vi "3dtest.vi"() -> ()   [LabVIEW 2022 SP3]
panel:
  in  "Planes to insert":u8=1
  in  "Save to File?":bool
  out "Array":u8[][][](array[numeric])
  in  "8-bit pixmap":u8[][][](array[numeric])=array17x236x252[1011024 elements]
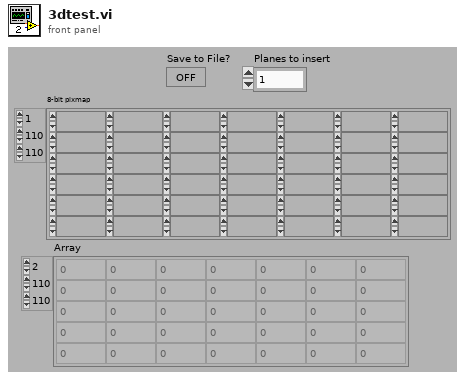
[diagram p1: front panel]
types:
  T1 = enum16{"open", "open or create", "create or replace", "create"}
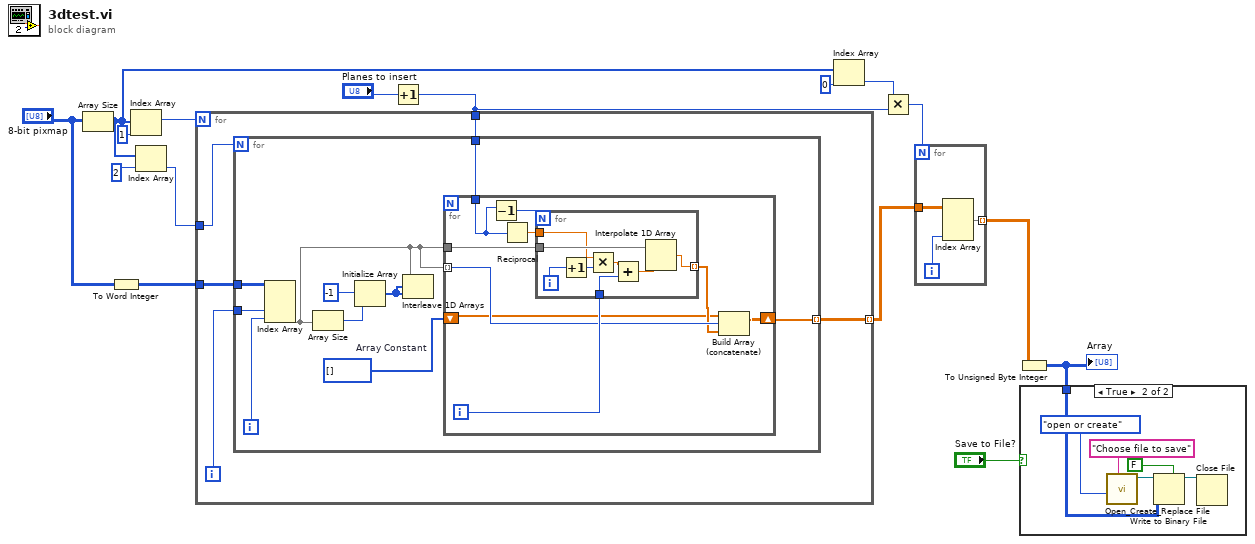
[diagram p0: block diagram]
diagram:
  n1 = Array Size(array="8-bit pixmap") -> (size(s)=w9:i32[])
  n2 = To Word Integer(number="8-bit pixmap") -> (16bit integer=w11:i16[][][])
  n3 = Index Array(array=w9, index=1) -> (element=w16:i32)
  n4 = Index Array(array=w9, index=2) -> (element=w15:i32)
  n5 = Increment(x="Planes to insert") -> (x+1=w1:u8)
  n6 = for {
    N: w16 -> [_]
    tunnel: w15 -> [w21]
    tunnel: w11 -> [w20]
    tunnel: [w18] -> w6 mode=indexing
    tunnel: w1 -> [w17]
    i -> [w19]
    n7 = for {
      N: w21 -> [_]
      tunnel: w20 -> [w31]
      tunnel: w19 -> [w30]
      tunnel: [w23] -> w18 mode=indexing
      tunnel: w17 -> [w22]
      i -> [w29]
      w24 = i16[] []  # Array Constant
      n8 = Index Array(array=w31, index (dim 1)=w30, index (dim 2)=w29) -> (element=w25:i16[])  [unwired: 1 in]
      n9 = Array Size(array=w25) -> (size(s)=w26:i32)
      n10 = Initialize Array(-1, w26) -> (w28:i32[])
      n11 = Interleave 1D Arrays(w25, w28, w28) -> ()  [unwired: 1 out]
      n12 = for {
        tunnel: w25 -> [w38]
        tunnel: w25 -> [w37] mode=indexing
        shift-right: [w35] -> w23
        shift-left: w24 -> [w34]
        tunnel: w22 -> [w33]
        i -> [w40]
        n13 = Decrement(x=w33) -> (x-1=w32:u8)
        n14 = Reciprocal(x=w33) -> (1/x=w39:dbl)
        n15 = for {
          N: w32 -> [_]
          tunnel: w40 -> [w43]
          tunnel: w39 -> [w44]
          tunnel: w38 -> [w48]
          tunnel: [w47] -> w36 mode=indexing
          i -> [w46]
          n16 = Increment(x=w46) -> (x+1=w45:i32)
          n17 = Multiply(x=w44, y=w45) -> (x*y=w42:dbl)
          n18 = Add(x=w42, y=w43) -> (x+y=w41:dbl)
          n19 = Interpolate 1D Array(1:w41, 2:w48) -> (0:w47:dbl)
        }
        n20 = Build Array (concatenate)(w34, w37, w36) -> (w35:dbl[])
      }
    }
  }
  n21 = Index Array(array=w9, index=0) -> (element=w8:i32)
  n22 = Multiply(x=w8, y=w1) -> (x*y=w7:i32)
  n23 = for {
    N: w7 -> [_]
    tunnel: w6 -> [w51]
    tunnel: [w49] -> w5 mode=indexing
    i -> [w50]
    n24 = Index Array(array=w51, index (dim 2)=w50) -> (element=w49:dbl[][])  [unwired: 2 in]
  }
  n25 = To Unsigned Byte Integer(number=w5) -> (unsigned 8bit integer=w4:u8[][][])
  "Array" <- w4
  n26 = case shown="True" "Save to File?" {
    tunnel: w4 -> [_ w53]
    frame False {
    }
    frame True {
      n27 = call <vilib>:"Open_Create_Replace File.vi"("prompt"="Choose file to save", "function (open:0)"=T1."open or create") -> ("refnum"=w57:refnum<file>)  [unwired: 4 in, 5 out]
      n28 = Write to Binary File(file (use dialog)=w57, data=w53, 5:FALSE ("prepend array or string size? (T)")) -> (refnum out=w56:refnum<file>)  [unwired: 1 in, 4 out]
      n29 = Close File(refnum=w56) -> ()  [unwired: 1 in, 2 out]
    }
  }
